vi "DigitalINStatus.vi"(8 "error in (no error)":errorcluster caption="错误输入（无错误）", 11 "handle":u64) -> (0 "error out":errorcluster caption="错误输出", 1 "status":i32=2, 2 "function return":i32, 3 "handle out":u64)   [LabVIEW 2018]
doc: "Set pos. or neg. Supply voltage"
uses:
  InstrumentsPlayground.lvlib
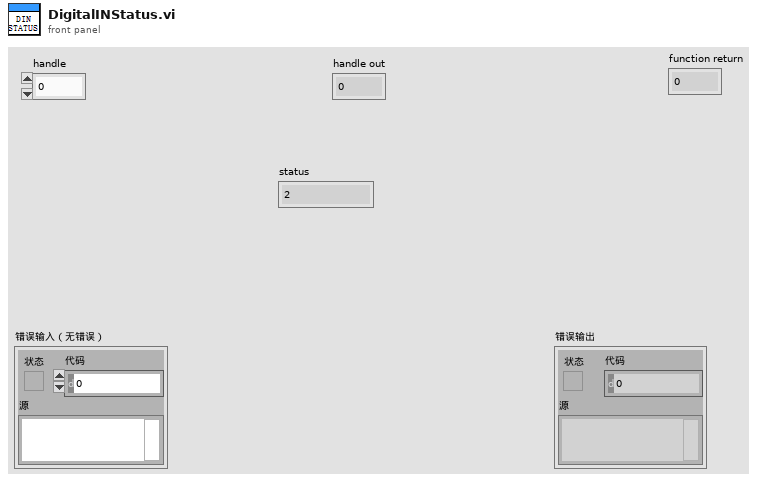
[diagram p1: front panel]
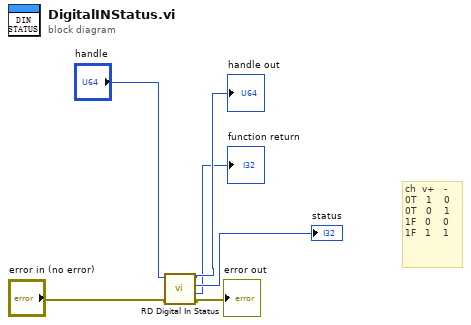
[diagram p0: block diagram]
diagram:
  # "ch  v+   -\n0T   1    0\n0T   0    1\n1F   0    0\n1F   1    1"
  n1 = call "RD Digital In Status.vi"("error in (no error)"="error in (no error)", "handle"="handle") -> ("error out"=→"error out":errorcluster, "function return"=→"function return":i32, "sts out"=→"status":u8, "handle out"=→"handle out":u64)  [unwired: 6 in]
